vi "write_access_codes_to_file.vi"(8 "error in":errorcluster, 10 "Codes":T2, 11 "Paths In":T1) -> (0 "error out":errorcluster)   [LabVIEW 2016]
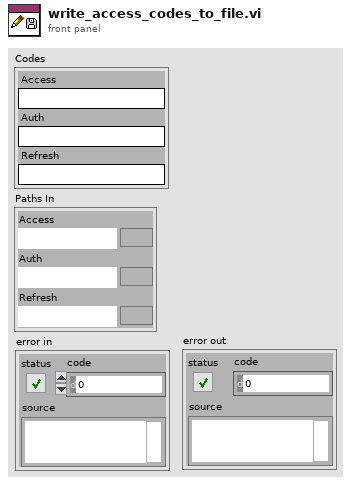
[diagram p1: front panel]
types:
  T1 = cluster{"Access":path, "Auth":path, "Refresh":path}
  T2 = cluster{"Access":string, "Auth":string, "Refresh":string}
  T3 = enum16{"open", "replace", "create", "open or create", "replace or create", "replace or create with confirmation"}
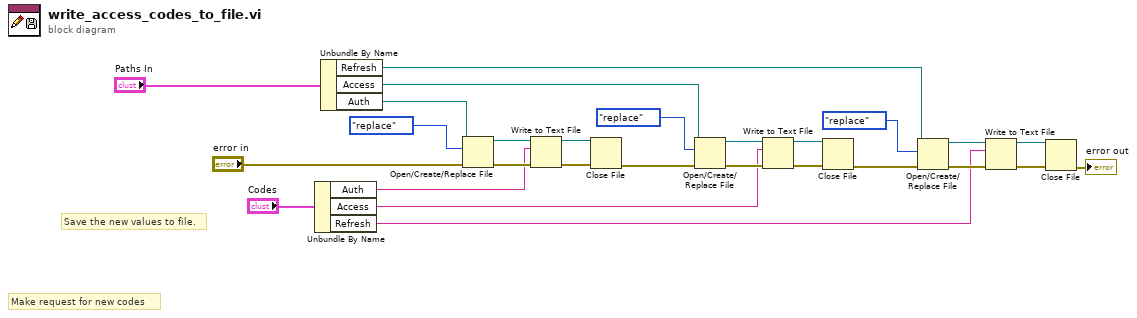
[diagram p0: block diagram]
diagram:
  # "Save the new values to file."
  # "Make request for new codes"
  n1 = Unbundle By Name("Codes") -> ("Auth"=w6:string, "Access"=w7:string, "Refresh"=w8:string)
  n2 = Unbundle By Name("Paths In") -> ("Refresh"=w10:path, "Access"=w13:path, "Auth"=w11:path)
  n3 = Open/Create/Replace File(file path (use dialog)=w11, error in="error in", operation (0:open)=T3."replace") -> (refnum out=w20:refnum<file>, error out=w22:errorcluster)  [unwired: 3 in, 1 out]
  n4 = Write to Text File(file (use dialog)=w20, text=w6, error in=w22) -> (refnum out=w21:refnum<file>, error out=w23:errorcluster)  [unwired: 1 in, 1 out]
  n5 = Close File(refnum=w21, error in=w23) -> (error out=w12:errorcluster)  [unwired: 1 out]
  n6 = Open/Create/Replace File(file path (use dialog)=w13, error in=w12, operation (0:open)=T3."replace") -> (refnum out=w27:refnum<file>, error out=w25:errorcluster)  [unwired: 3 in, 1 out]
  n7 = Write to Text File(file (use dialog)=w27, text=w7, error in=w25) -> (refnum out=w26:refnum<file>, error out=w24:errorcluster)  [unwired: 1 in, 1 out]
  n8 = Close File(refnum=w26, error in=w24) -> (error out=w9:errorcluster)  [unwired: 1 out]
  n9 = Open/Create/Replace File(file path (use dialog)=w10, error in=w9, operation (0:open)=T3."replace") -> (refnum out=w16:refnum<file>, error out=w18:errorcluster)  [unwired: 3 in, 1 out]
  n10 = Write to Text File(file (use dialog)=w16, text=w8, error in=w18) -> (refnum out=w17:refnum<file>, error out=w19:errorcluster)  [unwired: 1 in, 1 out]
  n11 = Close File(refnum=w17, error in=w19) -> (error out=→"error out":errorcluster)  [unwired: 1 out]
